vi "PotTempVI-Version3-2009.vi"() -> ()   [LabVIEW 2009]
uses:
  C/Program Files (x86)/National Instruments/LabVIEW 2014/instr.lib/Lake Shore Cryotronics 370/Lake Shore Cryotronics 370.lvlib
panel:
  in  "File Path":path
  out "Cernox Temperature 2":dbl
  out "Cernox Temperature 1":dbl
  out "Cernox Temperature 3":dbl
  out "Channel 3":cluster{dbl[], dbl[]}(graph)
  out "Channel 2":cluster{dbl[], dbl[]}(graph)
  out "Channel 1":cluster{dbl[], dbl[]}(graph)
  in  "CH1                CH2                Ch3":bool[](array[boolean])
  in  "Heater Range":u16(ring) items=["Off", "31.6 uA", "100 uA", "316 uA", "1.00 mA", "3.16 mA", "10.0 mA", "31.6 mA", "100 mA"]
  in  "Manual Output (0.000%)":dbl format="%#_13g"
  in  "(min)":dbl
  in  "(sec)":dbl
  in  "stop":bool
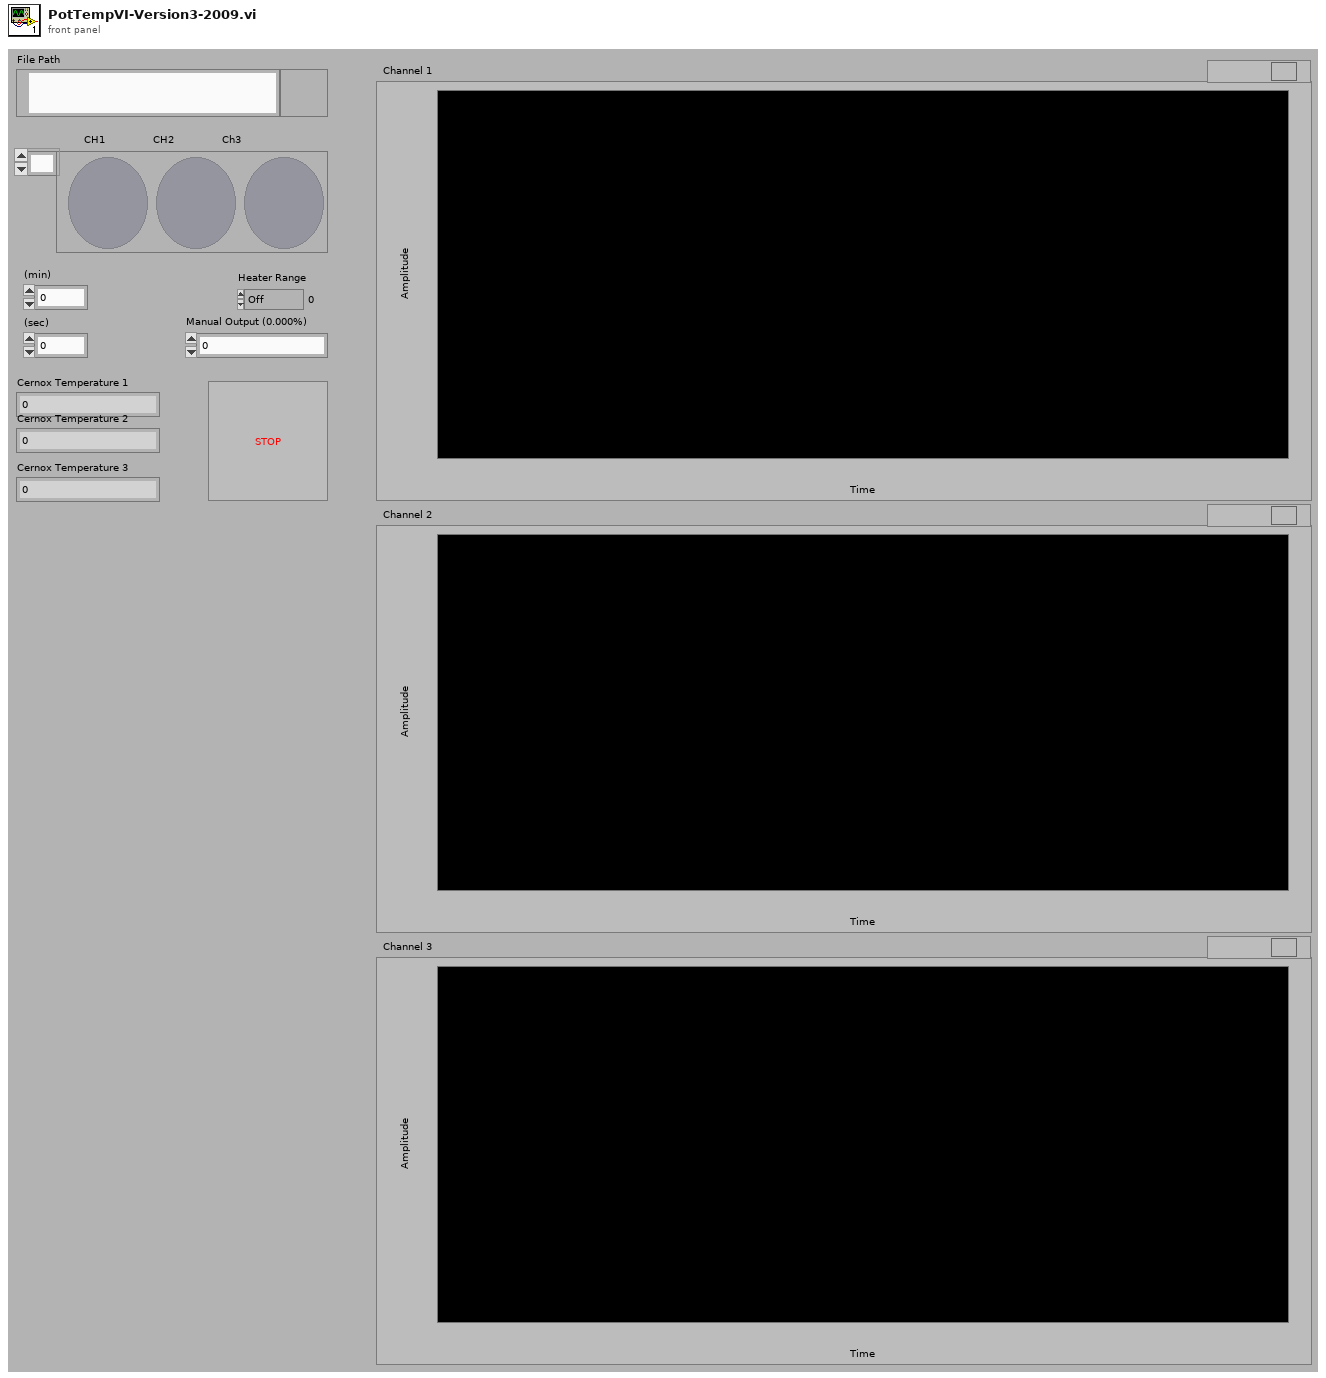
[diagram p1: front panel]
types:
  T1 = enum16{"open", "replace", "create", "open or create", "replace or create", "replace or create with confirmation"}
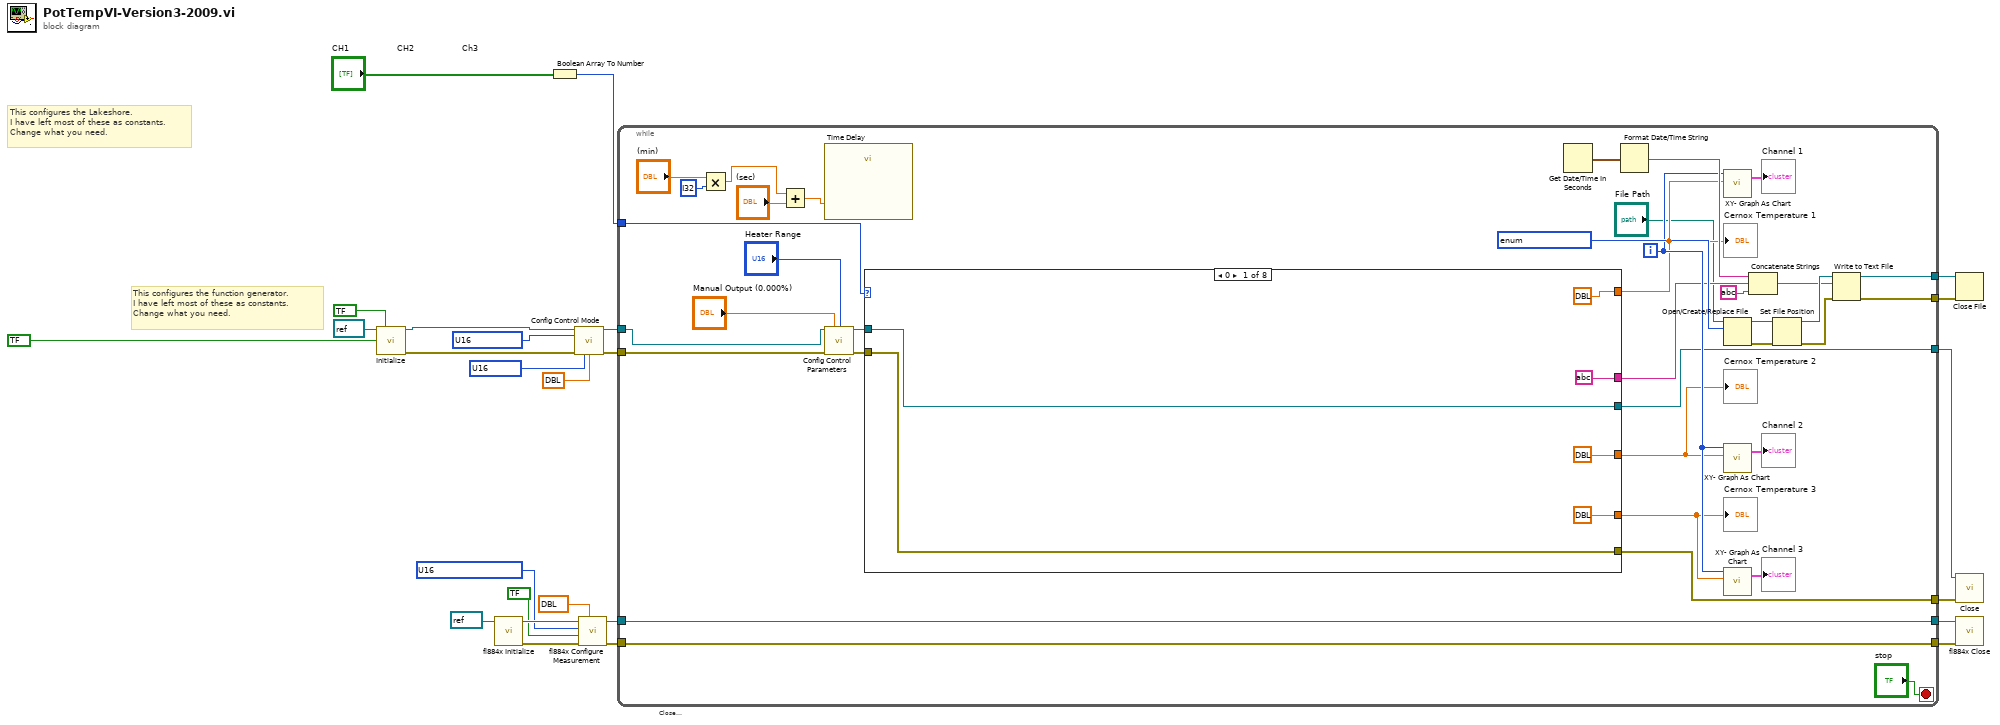
[diagram p0: block diagram]
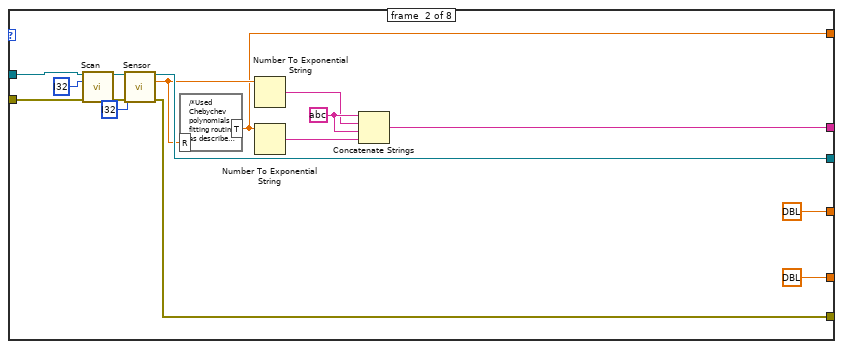
[diagram p2: hidden frame]
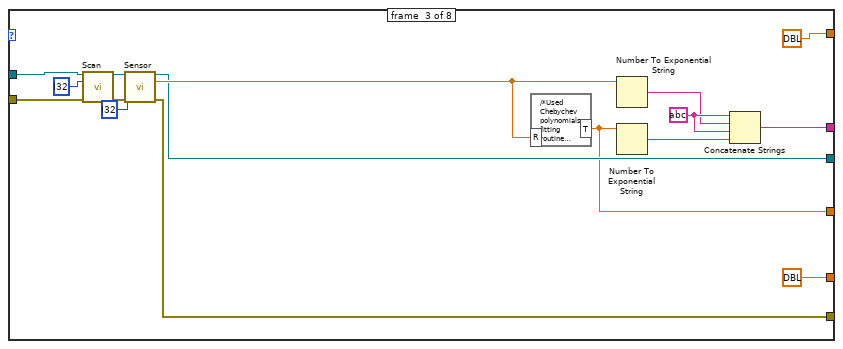
[diagram p3: hidden frame]
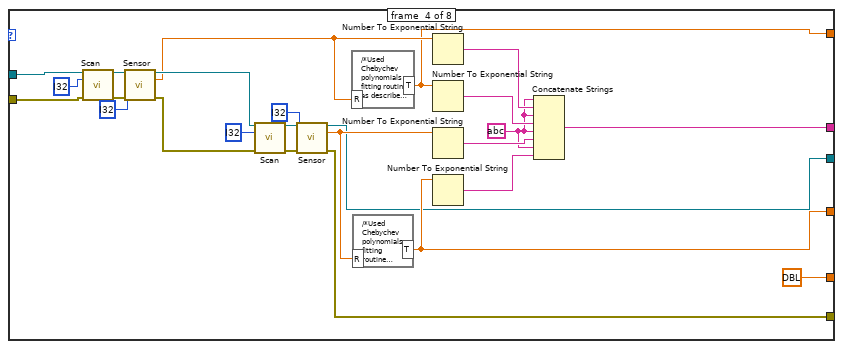
[diagram p4: hidden frame]
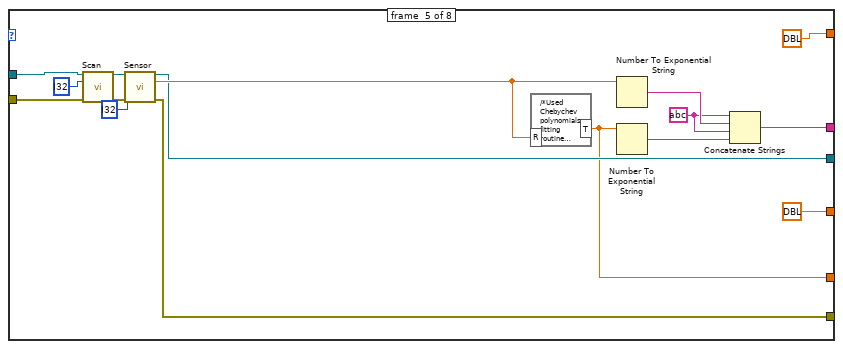
[diagram p5: hidden frame]
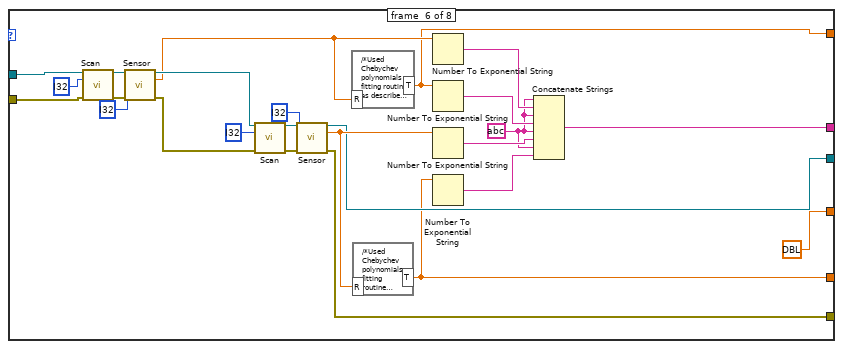
[diagram p6: hidden frame]
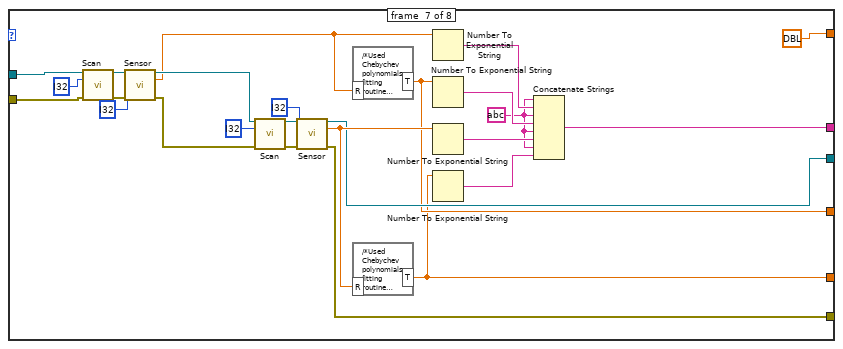
[diagram p7: hidden frame]
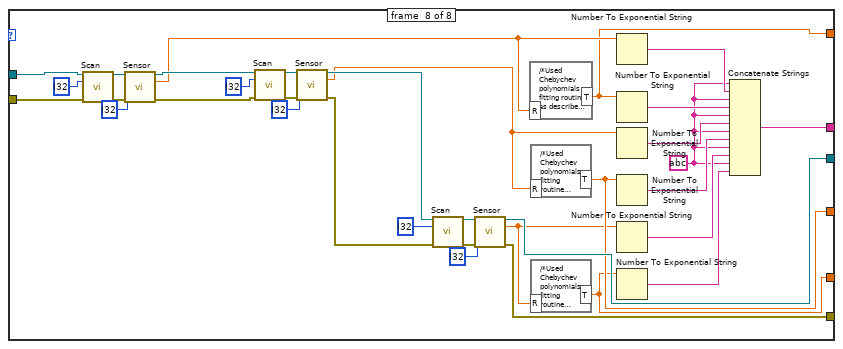
[diagram p8: hidden frame]
diagram:
  w7 = u16 ? items=["Current", "Power"] ("Heater Output Display (0: Current)")
  w9 = u16 ? items=["Closed Loop PID", "Zone Tuning", "Open Loop", "Off"] ("Control Mode (0: Closed Loop PID)")
  w23 = dbl ? items=["4.5", "5.5", "6.5"] ("Manual Resolution (5.5 Digits)")
  w24 = u16 ? items=["DC Voltage", "AC Voltage", "2 - Wire Resistance", "4 - Wire Resistance", "DC Current", "AC Current", "Frequency", "Period", "Continuity", "Diode Checking", "Temperature", "Capacitance"] ("Function (0: DC Voltage)")
  # "This configures the Lakeshore.\nI have left most of these as constants.\nChange what you need."
  # "This configures the function generator.\nI have left most of these as constants.\nChange what you need."
  # "Close Instrument."
  n1 = call "Initialize.vi"("VISA resource name"=refnum<visa-resource-name> ? ("VISA Resource Name 2"), "Reset to Default (False)"=bool ?, "Reset (True)"=bool ?) -> ("VISA resource name out"=w11:refnum<visa-resource-name>, "error out"=w10:errorcluster)  [unwired: 11 in]
  n2 = call "fl884x Initialize.vi"("VISA resource name"=refnum<visa-resource-name> ? ("VISA Resource Name")) -> ("error out"=w25:errorcluster, "VISA resource name out"=w26:refnum<visa-resource-name>)  [unwired: 9 in]
  n3 = Boolean Array To Number(Boolean array="CH1                CH2                Ch3") -> (number=w1:u32)
  n4 = call "Config Control Mode.vi"("VISA resource name"=w11, "Control Mode (0: Closed Loop PID)"=w9, "error in (no error)"=w10, "Heater Output Display (0: Current)"=w7, "Heater Resistance (100.00)"=dbl ?) -> ("VISA resource name out"=w6:refnum<visa-resource-name>, "error out"=w5:errorcluster)  [unwired: 9 in]
  n5 = call "fl884x Configure Measurement.vi"("Manual Resolution (5.5 Digits)"=w23, "error in (no error)"=w25, "Auto Range (T:Enable)"=bool ?, "Function (0: DC Voltage)"=w24, "VISA resource name"=w26) -> ("error out"=w19:errorcluster, "VISA resource name out"=w20:refnum<visa-resource-name>)  [unwired: 5 in]
  n6 = while {
    tunnel: w20 -> [w49]
    tunnel: w19 -> [w48]
    tunnel: w6 -> [w47]
    tunnel: w5 -> [w46]
    tunnel: [w49] -> w15
    tunnel: [w48] -> w18
    tunnel: [w56] -> w17
    tunnel: [w55] -> w16
    tunnel: [w35] -> w4
    tunnel: [w34] -> w3
    tunnel: w1 -> [w41]
    i -> [w36]
    stop <- "stop" stop-if-true
    n7 = Multiply(x="(min)", y=i32 ?) -> (x*y=w53:dbl)
    n8 = Add(x=w53, y="(sec)") -> (x+y=w52:dbl)
    n9 = call "Time Delay"("Delay Time (s)"=w52) -> ()  [unwired: 10 in, 1 out]
    n10 = call "Config Control Parameters.vi"("VISA resource name"=w47, "Manual Output (0.000%)"="Manual Output (0.000%)", "Heater Range (0: Off)"="Heater Range", "error in (no error)"=w46) -> ("VISA resource name out"=w40:refnum<visa-resource-name>, "error out"=w39:errorcluster)  [unwired: 10 in]
    n11 = case shown="0" w41 {
      tunnel: w40 -> [w69 w77 w93 w109 w135 w147 w174 w226]
      tunnel: w39 -> [w68 w76 w92 w108 w134 w151 w173 w225]
      tunnel: [dbl ? w71 dbl ? w104 dbl ? w145 dbl ? w197] -> w32
      tunnel: [w69 w79 w91 w107 w137 w156 w178 w214] -> w35
      tunnel: [w68 w78 w90 w106 w136 w150 w177 w213] -> w34
      tunnel: [dbl ? dbl ? w87 w110 dbl ? dbl ? w172 w206] -> w31
      tunnel: [dbl ? dbl ? dbl ? dbl ? w131 w153 w171 w202] -> w30
      tunnel: [string ? w75 w94 w112 w130 w154 w175 w199] -> w29
      frame #0 {
      }
      frame #1 {
        w85 = string ?
        n12 = call "Scan.vi"("VISA resource name"=w77, "Scan Channel (1)"=i32 ?, "error in (no error)"=w76) -> ("VISA resource name out"=w80:refnum<visa-resource-name>, "error out"=w82:errorcluster)  [unwired: 11 in]
        n13 = call "Sensor.vi"("VISA resource name"=w80, "Channel (1)"=i32 ?, "error in (no error)"=w82) -> ("VISA resource name out"=w79:refnum<visa-resource-name>, "Resistance Reading"=w72:dbl, "error out"=w78:errorcluster)  [unwired: 8 in, 2 out]
        n14 = formula code="/*Used Chebychev polynomials fitting routine\nas described in Calibration Report Description \ndocument. For future use with other thermometer, \njust replace, in all the appropriate\nranges, the Chebychev coefficients (array 'A[i]'), \nthe lower and upper boundaries for Z (variables 'ZU' \nand 'ZL'), and the numberof polynomial terms or \nfit range (variable 'range'). This information is \nfound in the data file for the corresponding \nthermometer */\n\n/*Declare variables. Used same notation\nas Lakeshore Calibration Report Description*/\n\nfloat64 Z, ZL, ZU, X, T;\nfloat64 Tc[12], A[12];\nint range, i;\nZ=log(R);\n\n\n/*Fit range 3, for R between 122.7738 and\n379.0544*/\nif(R>122.7738 && R<=379.0544)\n{\nrange=7;\nZL= 2.06767500767592;\nZU= 2.62579727581576;\nX=((Z-ZL)-(ZU-Z))/(ZU-ZL);\nA[0]=5.89345488289531E+00;\nA[1]=-6.65662879806624E+00;\nA[2]=2.58839377481062E+00;\nA[3]=-7.79761085327563E-01;\nA[4]=1.81747664835559E-01;\nA[5]=-2.85948965899305E-02;\nA[6]=3.14756394066286E-04;\nA[7]=1.58182677797188E-03;\nA[8]=-1.62769128118703E-03;\n\nTc[0]=1;\nTc[1]=X;\nT=A[0]+A[1]*X;\n\nfor(i=2; i<=range; i++)\n{\nTc[i]=2*X*Tc[i-1]-Tc[i-2];\nT=T+Tc[i]*A[i];\n}\n}\n\n/*Fit range 2, for R between 59.7368 and\n122.7738*/\nif(R> 59.7368 && R<=122.7738)\n{\nrange=7;\nZL= 1.75200116332745;\nZU= 2.11435743095945;\nX=((Z-ZL)-(ZU-Z))/(ZU-ZL);\nA[0]=4.32234727947262E+01;\nA[1]=-3.81351999747578E+01;\nA[2]=7.81449116299263E+00;\nA[3]=-8.59375474039158E-01;\nA[4]= 1.00417492862823E-01;\nA[5]=1.74498449889679E-03;\nA[6]=-1.20713645610291E-02;\nA[7]=1.63447339264850E-03;\n\nTc[0]=1;\nTc[1]=X;\nT=A[0]+A[1]*X;\n\nfor(i=2; i<=range; i++)\n{\nTc[i]=2*X*Tc[i-1]-Tc[i-2];\nT=T+Tc[i]*A[i];\n}\n}\n\n/*Fit range 1, for R between 28.7437 and\n8273.0144*/\nif(R> 28.7437 && R<=59.7368)\n{\nrange=7;\nZL= 1.45494394005744;\nZU= 1.80316018562455;\nX=((Z-ZL)-(ZU-Z))/(ZU-ZL);\nA[0]=1.78354115735659E+02;\nA[1]=-1.26988903132178E+02;\nA[2]=2.11414551345279E+01;\nA[3]=-2.87039950284064E+00;\nA[4]= 6.30799574782896E-01;\nA[5]=-1.42209214015529E-01;\nA[6]=3.09622419372907E-02;\nA[7]=-9.63520999389506E-03;\n\nTc[0]=1;\nTc[1]=X;\nT=A[0]+A[1]*X;\n\nfor(i=2; i<=range; i++)\n{\nTc[i]=2*X*Tc[i-1]-Tc[i-2];\nT=T+Tc[i]*A[i];\n}\n}"("R"=w72) -> ("T"=w71:dbl)
        n15 = Number To Exponential String(number=w72) -> (E-format string=w83:string)  [unwired: 3 in]
        n16 = Number To Exponential String(number=w71) -> (E-format string=w84:string)  [unwired: 3 in]
        n17 = Concatenate Strings(w85, w83, w85, w84) -> (w75:string)
      }
      frame #2 {
        w101 = string ?
        n18 = call "Scan.vi"("VISA resource name"=w93, "Scan Channel (1)"=i32 ?, "error in (no error)"=w92) -> ("VISA resource name out"=w95:refnum<visa-resource-name>, "error out"=w97:errorcluster)  [unwired: 11 in]
        n19 = call "Sensor.vi"("VISA resource name"=w95, "Channel (1)"=i32 ?, "error in (no error)"=w97) -> ("VISA resource name out"=w91:refnum<visa-resource-name>, "Resistance Reading"=w98:dbl, "error out"=w90:errorcluster)  [unwired: 8 in, 2 out]
        n20 = formula code="/*Used Chebychev polynomials fitting routine\nas described in Calibration Report Description \ndocument. For future use with other thermometer, \njust replace, in all the appropriate\nranges, the Chebychev coefficients (array 'A[i]'), \nthe lower and upper boundaries for Z (variables 'ZU' \nand 'ZL'), and the numberof polynomial terms or \nfit range (variable 'range'). This information is \nfound in the data file for the corresponding \nthermometer */\n\n/*Declare variables. Used same notation\nas Lakeshore Calibration Report Description*/\n\nfloat64 Z, ZL, ZU, X, T;\nfloat64 Tc[12], A[12];\nint range, i;\nZ=log(R);\n\n/*Fit range 4, for R between 27.8145 and\n55.2018*/\nif(R>=27.8145 && R<=55.2018)\n{\nrange=7;\nZL= 1.44074353015701;\nZU=1.76670659886134;\nX=((Z-ZL)-(ZU-Z))/(ZU-ZL);\nA[0]=1.82158062367373E+02;\nA[1]=-1.24663785394699E+02;\nA[2]= 1.99707471344437E+01;\nA[3]=-2.68638755066500E+00;\nA[4]=5.62902207096738E-01;\nA[5]= -1.04899492331528E-01;\nA[6]=1.47394426824740E-02;\nA[7]=-1.09663024188992E-02;\n\nTc[0]=1;\nTc[1]=X;\nT=A[0]+A[1]*X;\n\nfor(i=2; i<=range; i++)\n{\nTc[i]=2*X*Tc[i-1]-Tc[i-2];\nT=T+Tc[i]*A[i];\n}\n}\n\n/*Fit range 3, for R between 55.2018 and\n111.4842*/\nif(R>55.2018 && R<=111.4842)\n{\nrange=9;\nZL= 1.71936458773677;\nZU= 2.06940247551414;\nX=((Z-ZL)-(ZU-Z))/(ZU-ZL);\nA[0]=4.61222264729901E+01;\nA[1]=-4.01018177367225E+01;\nA[2]=8.04410401028361E+00;\nA[3]=-8.87825177741193E-01;\nA[4]= 9.46412812559081E-02;\nA[5]=1.14695723765652E-02;\nA[6]=-1.28476433375258E-02;\nA[7]=2.61003207902573E-03;\nA[8]=-1.62769128118703E-03;\nA[9]=2.14879733652881E-03;\n\nTc[0]=1;\nTc[1]=X;\nT=A[0]+A[1]*X;\n\nfor(i=2; i<=range; i++)\n{\nTc[i]=2*X*Tc[i-1]-Tc[i-2];\nT=T+Tc[i]*A[i];\n}\n}\n\n/*Fit range 2, for R between 111.4842 and\n313.6289*/\nif(R> 111.4842 && R<=313.6289)\n{\nrange=8;\nZL= 2.02806379707861;\nZU= 2.55512620740659;\nX=((Z-ZL)-(ZU-Z))/(ZU-ZL);\nA[0]=6.35009482366579E+00;\nA[1]=-7.12992063705802E+00;\nA[2]=2.72290509023981E+00;\nA[3]=-7.95127185574136E-01;\nA[4]= 1.75501651647015E-01;\nA[5]=-2.36820706103904E-02;\nA[6]=-1.48683367592906E-03;\nA[7]=2.20400453630561E-03;\nA[8]=-7.29658382785940E-04;\n\nTc[0]=1;\nTc[1]=X;\nT=A[0]+A[1]*X;\n\nfor(i=2; i<=range; i++)\n{\nTc[i]=2*X*Tc[i-1]-Tc[i-2];\nT=T+Tc[i]*A[i];\n}\n}\n\n/*Fit range 1, for R between 313.6289 and\n8273.0144*/\nif(R>  313.6289 && R<=8273.0144)\n{\nrange=11;\nZL= 2.43768275202674;\nZU= 4.08120684160154;\nX=((Z-ZL)-(ZU-Z))/(ZU-ZL);\nA[0]=5.67750174822212E-01;\nA[1]=-7.48399352555430E-01;\nA[2]=3.88178435547519E-01;\nA[3]=-1.77340445603059E-01;\nA[4]= 7.34297995027544E-02;\nA[5]=-2.89170333461975E-02;\nA[6]=1.12452775189607E-02;\nA[7]=-3.77083878348011E-03;\nA[8]=1.58754722583042E-03;\nA[9]=-1.76346768933995E-04;\nA[10]=4.11858083918786E-04;\nA[11]=3.67394984257076E-04;\n\nTc[0]=1;\nTc[1]=X;\nT=A[0]+A[1]*X;\n\nfor(i=2; i<=range; i++)\n{\nTc[i]=2*X*Tc[i-1]-Tc[i-2];\nT=T+Tc[i]*A[i];\n}\n}"("R"=w98) -> ("T"=w87:dbl)
        n21 = Number To Exponential String(number=w98) -> (E-format string=w99:string)  [unwired: 3 in]
        n22 = Number To Exponential String(number=w87) -> (E-format string=w100:string)  [unwired: 3 in]
        n23 = Concatenate Strings(w101, w99, w101, w100) -> (w94:string)
      }
      frame #3 {
        w111 = string ?
        n24 = call "Scan.vi"("VISA resource name"=w109, "Scan Channel (1)"=i32 ?, "error in (no error)"=w108) -> ("VISA resource name out"=w125:refnum<visa-resource-name>, "error out"=w124:errorcluster)  [unwired: 11 in]
        n25 = call "Sensor.vi"("VISA resource name"=w125, "Channel (1)"=i32 ?, "error in (no error)"=w124) -> ("VISA resource name out"=w122:refnum<visa-resource-name>, "Resistance Reading"=w105:dbl, "error out"=w121:errorcluster)  [unwired: 8 in, 2 out]
        n26 = call "Scan.vi"("VISA resource name"=w122, "Scan Channel (1)"=i32 ?, "error in (no error)"=w121) -> ("VISA resource name out"=w123:refnum<visa-resource-name>, "error out"=w119:errorcluster)  [unwired: 11 in]
        n27 = call "Sensor.vi"("VISA resource name"=w123, "Channel (1)"=i32 ?, "error in (no error)"=w119) -> ("VISA resource name out"=w107:refnum<visa-resource-name>, "Resistance Reading"=w116:dbl, "error out"=w106:errorcluster)  [unwired: 8 in, 2 out]
        n28 = formula code="/*Used Chebychev polynomials fitting routine\nas described in Calibration Report Description \ndocument. For future use with other thermometer, \njust replace, in all the appropriate\nranges, the Chebychev coefficients (array 'A[i]'), \nthe lower and upper boundaries for Z (variables 'ZU' \nand 'ZL'), and the numberof polynomial terms or \nfit range (variable 'range'). This information is \nfound in the data file for the corresponding \nthermometer */\n\n/*Declare variables. Used same notation\nas Lakeshore Calibration Report Description*/\n\nfloat64 Z, ZL, ZU, X, T;\nfloat64 Tc[12], A[12];\nint range, i;\nZ=log(R);\n\n\n/*Fit range 3, for R between 122.7738 and\n379.0544*/\nif(R>122.7738 && R<=379.0544)\n{\nrange=7;\nZL= 2.06767500767592;\nZU= 2.62579727581576;\nX=((Z-ZL)-(ZU-Z))/(ZU-ZL);\nA[0]=5.89345488289531E+00;\nA[1]=-6.65662879806624E+00;\nA[2]=2.58839377481062E+00;\nA[3]=-7.79761085327563E-01;\nA[4]=1.81747664835559E-01;\nA[5]=-2.85948965899305E-02;\nA[6]=3.14756394066286E-04;\nA[7]=1.58182677797188E-03;\nA[8]=-1.62769128118703E-03;\n\nTc[0]=1;\nTc[1]=X;\nT=A[0]+A[1]*X;\n\nfor(i=2; i<=range; i++)\n{\nTc[i]=2*X*Tc[i-1]-Tc[i-2];\nT=T+Tc[i]*A[i];\n}\n}\n\n/*Fit range 2, for R between 59.7368 and\n122.7738*/\nif(R> 59.7368 && R<=122.7738)\n{\nrange=7;\nZL= 1.75200116332745;\nZU= 2.11435743095945;\nX=((Z-ZL)-(ZU-Z))/(ZU-ZL);\nA[0]=4.32234727947262E+01;\nA[1]=-3.81351999747578E+01;\nA[2]=7.81449116299263E+00;\nA[3]=-8.59375474039158E-01;\nA[4]= 1.00417492862823E-01;\nA[5]=1.74498449889679E-03;\nA[6]=-1.20713645610291E-02;\nA[7]=1.63447339264850E-03;\n\nTc[0]=1;\nTc[1]=X;\nT=A[0]+A[1]*X;\n\nfor(i=2; i<=range; i++)\n{\nTc[i]=2*X*Tc[i-1]-Tc[i-2];\nT=T+Tc[i]*A[i];\n}\n}\n\n/*Fit range 1, for R between 28.7437 and\n8273.0144*/\nif(R> 28.7437 && R<=59.7368)\n{\nrange=7;\nZL= 1.45494394005744;\nZU= 1.80316018562455;\nX=((Z-ZL)-(ZU-Z))/(ZU-ZL);\nA[0]=1.78354115735659E+02;\nA[1]=-1.26988903132178E+02;\nA[2]=2.11414551345279E+01;\nA[3]=-2.87039950284064E+00;\nA[4]= 6.30799574782896E-01;\nA[5]=-1.42209214015529E-01;\nA[6]=3.09622419372907E-02;\nA[7]=-9.63520999389506E-03;\n\nTc[0]=1;\nTc[1]=X;\nT=A[0]+A[1]*X;\n\nfor(i=2; i<=range; i++)\n{\nTc[i]=2*X*Tc[i-1]-Tc[i-2];\nT=T+Tc[i]*A[i];\n}\n}"("R"=w105) -> ("T"=w104:dbl)
        n29 = formula code="/*Used Chebychev polynomials fitting routine\nas described in Calibration Report Description \ndocument. For future use with other thermometer, \njust replace, in all the appropriate\nranges, the Chebychev coefficients (array 'A[i]'), \nthe lower and upper boundaries for Z (variables 'ZU' \nand 'ZL'), and the numberof polynomial terms or \nfit range (variable 'range'). This information is \nfound in the data file for the corresponding \nthermometer */\n\n/*Declare variables. Used same notation\nas Lakeshore Calibration Report Description*/\n\nfloat64 Z, ZL, ZU, X, T;\nfloat64 Tc[12], A[12];\nint range, i;\nZ=log(R);\n\n/*Fit range 4, for R between 27.8145 and\n55.2018*/\nif(R>=27.8145 && R<=55.2018)\n{\nrange=7;\nZL= 1.44074353015701;\nZU=1.76670659886134;\nX=((Z-ZL)-(ZU-Z))/(ZU-ZL);\nA[0]=1.82158062367373E+02;\nA[1]=-1.24663785394699E+02;\nA[2]= 1.99707471344437E+01;\nA[3]=-2.68638755066500E+00;\nA[4]=5.62902207096738E-01;\nA[5]= -1.04899492331528E-01;\nA[6]=1.47394426824740E-02;\nA[7]=-1.09663024188992E-02;\n\nTc[0]=1;\nTc[1]=X;\nT=A[0]+A[1]*X;\n\nfor(i=2; i<=range; i++)\n{\nTc[i]=2*X*Tc[i-1]-Tc[i-2];\nT=T+Tc[i]*A[i];\n}\n}\n\n/*Fit range 3, for R between 55.2018 and\n111.4842*/\nif(R>55.2018 && R<=111.4842)\n{\nrange=9;\nZL= 1.71936458773677;\nZU= 2.06940247551414;\nX=((Z-ZL)-(ZU-Z))/(ZU-ZL);\nA[0]=4.61222264729901E+01;\nA[1]=-4.01018177367225E+01;\nA[2]=8.04410401028361E+00;\nA[3]=-8.87825177741193E-01;\nA[4]= 9.46412812559081E-02;\nA[5]=1.14695723765652E-02;\nA[6]=-1.28476433375258E-02;\nA[7]=2.61003207902573E-03;\nA[8]=-1.62769128118703E-03;\nA[9]=2.14879733652881E-03;\n\nTc[0]=1;\nTc[1]=X;\nT=A[0]+A[1]*X;\n\nfor(i=2; i<=range; i++)\n{\nTc[i]=2*X*Tc[i-1]-Tc[i-2];\nT=T+Tc[i]*A[i];\n}\n}\n\n/*Fit range 2, for R between 111.4842 and\n313.6289*/\nif(R> 111.4842 && R<=313.6289)\n{\nrange=8;\nZL= 2.02806379707861;\nZU= 2.55512620740659;\nX=((Z-ZL)-(ZU-Z))/(ZU-ZL);\nA[0]=6.35009482366579E+00;\nA[1]=-7.12992063705802E+00;\nA[2]=2.72290509023981E+00;\nA[3]=-7.95127185574136E-01;\nA[4]= 1.75501651647015E-01;\nA[5]=-2.36820706103904E-02;\nA[6]=-1.48683367592906E-03;\nA[7]=2.20400453630561E-03;\nA[8]=-7.29658382785940E-04;\n\nTc[0]=1;\nTc[1]=X;\nT=A[0]+A[1]*X;\n\nfor(i=2; i<=range; i++)\n{\nTc[i]=2*X*Tc[i-1]-Tc[i-2];\nT=T+Tc[i]*A[i];\n}\n}\n\n/*Fit range 1, for R between 313.6289 and\n8273.0144*/\nif(R>  313.6289 && R<=8273.0144)\n{\nrange=11;\nZL= 2.43768275202674;\nZU= 4.08120684160154;\nX=((Z-ZL)-(ZU-Z))/(ZU-ZL);\nA[0]=5.67750174822212E-01;\nA[1]=-7.48399352555430E-01;\nA[2]=3.88178435547519E-01;\nA[3]=-1.77340445603059E-01;\nA[4]= 7.34297995027544E-02;\nA[5]=-2.89170333461975E-02;\nA[6]=1.12452775189607E-02;\nA[7]=-3.77083878348011E-03;\nA[8]=1.58754722583042E-03;\nA[9]=-1.76346768933995E-04;\nA[10]=4.11858083918786E-04;\nA[11]=3.67394984257076E-04;\n\nTc[0]=1;\nTc[1]=X;\nT=A[0]+A[1]*X;\n\nfor(i=2; i<=range; i++)\n{\nTc[i]=2*X*Tc[i-1]-Tc[i-2];\nT=T+Tc[i]*A[i];\n}\n}"("R"=w116) -> ("T"=w110:dbl)
        n30 = Number To Exponential String(number=w105) -> (E-format string=w118:string)  [unwired: 3 in]
        n31 = Number To Exponential String(number=w104) -> (E-format string=w117:string)  [unwired: 3 in]
        n32 = Number To Exponential String(number=w116) -> (E-format string=w115:string)  [unwired: 3 in]
        n33 = Number To Exponential String(number=w110) -> (E-format string=w114:string)  [unwired: 3 in]
        n34 = Concatenate Strings(w111, w118, w111, w117, w111, w115, w111, w114) -> (w112:string)
      }
      frame #4 {
        w128 = string ?
        n35 = call "Scan.vi"("VISA resource name"=w135, "Scan Channel (1)"=i32 ?, "error in (no error)"=w134) -> ("VISA resource name out"=w142:refnum<visa-resource-name>, "error out"=w140:errorcluster)  [unwired: 11 in]
        n36 = call "Sensor.vi"("VISA resource name"=w142, "Channel (1)"=i32 ?, "error in (no error)"=w140) -> ("VISA resource name out"=w137:refnum<visa-resource-name>, "Resistance Reading"=w139:dbl, "error out"=w136:errorcluster)  [unwired: 8 in, 2 out]
        n37 = formula code="/*Used Chebychev polynomials fitting routine\nas described in Calibration Report Description \ndocument. For future use with other thermometer, \njust replace, in all the appropriate\nranges, the Chebychev coefficients (array 'A[i]'), \nthe lower and upper boundaries for Z (variables 'ZU' \nand 'ZL'), and the numberof polynomial terms or \nfit range (variable 'range'). This information is \nfound in the data file for the corresponding \nthermometer */\n\n/*Declare variables. Used same notation\nas Lakeshore Calibration Report Description*/\n\nfloat64 Z, ZL, ZU, X, T;\nfloat64 Tc[12], A[12];\nint range, i;\nZ=log(R);\n\n/*Fit range 4, for R between 27.8145 and\n55.2018*/\nif(R>=27.8145 && R<=55.2018)\n{\nrange=7;\nZL= 1.44074353015701;\nZU=1.76670659886134;\nX=((Z-ZL)-(ZU-Z))/(ZU-ZL);\nA[0]=1.82158062367373E+02;\nA[1]=-1.24663785394699E+02;\nA[2]= 1.99707471344437E+01;\nA[3]=-2.68638755066500E+00;\nA[4]=5.62902207096738E-01;\nA[5]= -1.04899492331528E-01;\nA[6]=1.47394426824740E-02;\nA[7]=-1.09663024188992E-02;\n\nTc[0]=1;\nTc[1]=X;\nT=A[0]+A[1]*X;\n\nfor(i=2; i<=range; i++)\n{\nTc[i]=2*X*Tc[i-1]-Tc[i-2];\nT=T+Tc[i]*A[i];\n}\n}\n\n/*Fit range 3, for R between 55.2018 and\n111.4842*/\nif(R>55.2018 && R<=111.4842)\n{\nrange=9;\nZL= 1.71936458773677;\nZU= 2.06940247551414;\nX=((Z-ZL)-(ZU-Z))/(ZU-ZL);\nA[0]=4.61222264729901E+01;\nA[1]=-4.01018177367225E+01;\nA[2]=8.04410401028361E+00;\nA[3]=-8.87825177741193E-01;\nA[4]= 9.46412812559081E-02;\nA[5]=1.14695723765652E-02;\nA[6]=-1.28476433375258E-02;\nA[7]=2.61003207902573E-03;\nA[8]=-1.62769128118703E-03;\nA[9]=2.14879733652881E-03;\n\nTc[0]=1;\nTc[1]=X;\nT=A[0]+A[1]*X;\n\nfor(i=2; i<=range; i++)\n{\nTc[i]=2*X*Tc[i-1]-Tc[i-2];\nT=T+Tc[i]*A[i];\n}\n}\n\n/*Fit range 2, for R between 111.4842 and\n313.6289*/\nif(R> 111.4842 && R<=313.6289)\n{\nrange=8;\nZL= 2.02806379707861;\nZU= 2.55512620740659;\nX=((Z-ZL)-(ZU-Z))/(ZU-ZL);\nA[0]=6.35009482366579E+00;\nA[1]=-7.12992063705802E+00;\nA[2]=2.72290509023981E+00;\nA[3]=-7.95127185574136E-01;\nA[4]= 1.75501651647015E-01;\nA[5]=-2.36820706103904E-02;\nA[6]=-1.48683367592906E-03;\nA[7]=2.20400453630561E-03;\nA[8]=-7.29658382785940E-04;\n\nTc[0]=1;\nTc[1]=X;\nT=A[0]+A[1]*X;\n\nfor(i=2; i<=range; i++)\n{\nTc[i]=2*X*Tc[i-1]-Tc[i-2];\nT=T+Tc[i]*A[i];\n}\n}\n\n/*Fit range 1, for R between 313.6289 and\n8273.0144*/\nif(R>  313.6289 && R<=8273.0144)\n{\nrange=11;\nZL= 2.43768275202674;\nZU= 4.08120684160154;\nX=((Z-ZL)-(ZU-Z))/(ZU-ZL);\nA[0]=5.67750174822212E-01;\nA[1]=-7.48399352555430E-01;\nA[2]=3.88178435547519E-01;\nA[3]=-1.77340445603059E-01;\nA[4]= 7.34297995027544E-02;\nA[5]=-2.89170333461975E-02;\nA[6]=1.12452775189607E-02;\nA[7]=-3.77083878348011E-03;\nA[8]=1.58754722583042E-03;\nA[9]=-1.76346768933995E-04;\nA[10]=4.11858083918786E-04;\nA[11]=3.67394984257076E-04;\n\nTc[0]=1;\nTc[1]=X;\nT=A[0]+A[1]*X;\n\nfor(i=2; i<=range; i++)\n{\nTc[i]=2*X*Tc[i-1]-Tc[i-2];\nT=T+Tc[i]*A[i];\n}\n}"("R"=w139) -> ("T"=w131:dbl)
        n38 = Number To Exponential String(number=w139) -> (E-format string=w138:string)  [unwired: 3 in]
        n39 = Number To Exponential String(number=w131) -> (E-format string=w129:string)  [unwired: 3 in]
        n40 = Concatenate Strings(w128, w138, w128, w129) -> (w130:string)
      }
      frame #5 {
        w157 = string ?
        n41 = call "Scan.vi"("VISA resource name"=w147, "Scan Channel (1)"=i32 ?, "error in (no error)"=w151) -> ("VISA resource name out"=w166:refnum<visa-resource-name>, "error out"=w165:errorcluster)  [unwired: 11 in]
        n42 = call "Sensor.vi"("VISA resource name"=w166, "Channel (1)"=i32 ?, "error in (no error)"=w165) -> ("VISA resource name out"=w149:refnum<visa-resource-name>, "Resistance Reading"=w146:dbl, "error out"=w148:errorcluster)  [unwired: 8 in, 2 out]
        n43 = call "Scan.vi"("VISA resource name"=w149, "Scan Channel (1)"=i32 ?, "error in (no error)"=w148) -> ("VISA resource name out"=w164:refnum<visa-resource-name>, "error out"=w162:errorcluster)  [unwired: 11 in]
        n44 = call "Sensor.vi"("VISA resource name"=w164, "Channel (1)"=i32 ?, "error in (no error)"=w162) -> ("VISA resource name out"=w156:refnum<visa-resource-name>, "Resistance Reading"=w159:dbl, "error out"=w150:errorcluster)  [unwired: 8 in, 2 out]
        n45 = formula code="/*Used Chebychev polynomials fitting routine\nas described in Calibration Report Description \ndocument. For future use with other thermometer, \njust replace, in all the appropriate\nranges, the Chebychev coefficients (array 'A[i]'), \nthe lower and upper boundaries for Z (variables 'ZU' \nand 'ZL'), and the numberof polynomial terms or \nfit range (variable 'range'). This information is \nfound in the data file for the corresponding \nthermometer */\n\n/*Declare variables. Used same notation\nas Lakeshore Calibration Report Description*/\n\nfloat64 Z, ZL, ZU, X, T;\nfloat64 Tc[12], A[12];\nint range, i;\nZ=log(R);\n\n\n/*Fit range 3, for R between 122.7738 and\n379.0544*/\nif(R>122.7738 && R<=379.0544)\n{\nrange=7;\nZL= 2.06767500767592;\nZU= 2.62579727581576;\nX=((Z-ZL)-(ZU-Z))/(ZU-ZL);\nA[0]=5.89345488289531E+00;\nA[1]=-6.65662879806624E+00;\nA[2]=2.58839377481062E+00;\nA[3]=-7.79761085327563E-01;\nA[4]=1.81747664835559E-01;\nA[5]=-2.85948965899305E-02;\nA[6]=3.14756394066286E-04;\nA[7]=1.58182677797188E-03;\nA[8]=-1.62769128118703E-03;\n\nTc[0]=1;\nTc[1]=X;\nT=A[0]+A[1]*X;\n\nfor(i=2; i<=range; i++)\n{\nTc[i]=2*X*Tc[i-1]-Tc[i-2];\nT=T+Tc[i]*A[i];\n}\n}\n\n/*Fit range 2, for R between 59.7368 and\n122.7738*/\nif(R> 59.7368 && R<=122.7738)\n{\nrange=7;\nZL= 1.75200116332745;\nZU= 2.11435743095945;\nX=((Z-ZL)-(ZU-Z))/(ZU-ZL);\nA[0]=4.32234727947262E+01;\nA[1]=-3.81351999747578E+01;\nA[2]=7.81449116299263E+00;\nA[3]=-8.59375474039158E-01;\nA[4]= 1.00417492862823E-01;\nA[5]=1.74498449889679E-03;\nA[6]=-1.20713645610291E-02;\nA[7]=1.63447339264850E-03;\n\nTc[0]=1;\nTc[1]=X;\nT=A[0]+A[1]*X;\n\nfor(i=2; i<=range; i++)\n{\nTc[i]=2*X*Tc[i-1]-Tc[i-2];\nT=T+Tc[i]*A[i];\n}\n}\n\n/*Fit range 1, for R between 28.7437 and\n8273.0144*/\nif(R> 28.7437 && R<=59.7368)\n{\nrange=7;\nZL= 1.45494394005744;\nZU= 1.80316018562455;\nX=((Z-ZL)-(ZU-Z))/(ZU-ZL);\nA[0]=1.78354115735659E+02;\nA[1]=-1.26988903132178E+02;\nA[2]=2.11414551345279E+01;\nA[3]=-2.87039950284064E+00;\nA[4]= 6.30799574782896E-01;\nA[5]=-1.42209214015529E-01;\nA[6]=3.09622419372907E-02;\nA[7]=-9.63520999389506E-03;\n\nTc[0]=1;\nTc[1]=X;\nT=A[0]+A[1]*X;\n\nfor(i=2; i<=range; i++)\n{\nTc[i]=2*X*Tc[i-1]-Tc[i-2];\nT=T+Tc[i]*A[i];\n}\n}"("R"=w146) -> ("T"=w145:dbl)
        n46 = formula code="/*Used Chebychev polynomials fitting routine\nas described in Calibration Report Description \ndocument. For future use with other thermometer, \njust replace, in all the appropriate\nranges, the Chebychev coefficients (array 'A[i]'), \nthe lower and upper boundaries for Z (variables 'ZU' \nand 'ZL'), and the numberof polynomial terms or \nfit range (variable 'range'). This information is \nfound in the data file for the corresponding \nthermometer */\n\n/*Declare variables. Used same notation\nas Lakeshore Calibration Report Description*/\n\nfloat64 Z, ZL, ZU, X, T;\nfloat64 Tc[12], A[12];\nint range, i;\nZ=log(R);\n\n/*Fit range 4, for R between 27.8145 and\n55.2018*/\nif(R>=27.8145 && R<=55.2018)\n{\nrange=7;\nZL= 1.44074353015701;\nZU=1.76670659886134;\nX=((Z-ZL)-(ZU-Z))/(ZU-ZL);\nA[0]=1.82158062367373E+02;\nA[1]=-1.24663785394699E+02;\nA[2]= 1.99707471344437E+01;\nA[3]=-2.68638755066500E+00;\nA[4]=5.62902207096738E-01;\nA[5]= -1.04899492331528E-01;\nA[6]=1.47394426824740E-02;\nA[7]=-1.09663024188992E-02;\n\nTc[0]=1;\nTc[1]=X;\nT=A[0]+A[1]*X;\n\nfor(i=2; i<=range; i++)\n{\nTc[i]=2*X*Tc[i-1]-Tc[i-2];\nT=T+Tc[i]*A[i];\n}\n}\n\n/*Fit range 3, for R between 55.2018 and\n111.4842*/\nif(R>55.2018 && R<=111.4842)\n{\nrange=9;\nZL= 1.71936458773677;\nZU= 2.06940247551414;\nX=((Z-ZL)-(ZU-Z))/(ZU-ZL);\nA[0]=4.61222264729901E+01;\nA[1]=-4.01018177367225E+01;\nA[2]=8.04410401028361E+00;\nA[3]=-8.87825177741193E-01;\nA[4]= 9.46412812559081E-02;\nA[5]=1.14695723765652E-02;\nA[6]=-1.28476433375258E-02;\nA[7]=2.61003207902573E-03;\nA[8]=-1.62769128118703E-03;\nA[9]=2.14879733652881E-03;\n\nTc[0]=1;\nTc[1]=X;\nT=A[0]+A[1]*X;\n\nfor(i=2; i<=range; i++)\n{\nTc[i]=2*X*Tc[i-1]-Tc[i-2];\nT=T+Tc[i]*A[i];\n}\n}\n\n/*Fit range 2, for R between 111.4842 and\n313.6289*/\nif(R> 111.4842 && R<=313.6289)\n{\nrange=8;\nZL= 2.02806379707861;\nZU= 2.55512620740659;\nX=((Z-ZL)-(ZU-Z))/(ZU-ZL);\nA[0]=6.35009482366579E+00;\nA[1]=-7.12992063705802E+00;\nA[2]=2.72290509023981E+00;\nA[3]=-7.95127185574136E-01;\nA[4]= 1.75501651647015E-01;\nA[5]=-2.36820706103904E-02;\nA[6]=-1.48683367592906E-03;\nA[7]=2.20400453630561E-03;\nA[8]=-7.29658382785940E-04;\n\nTc[0]=1;\nTc[1]=X;\nT=A[0]+A[1]*X;\n\nfor(i=2; i<=range; i++)\n{\nTc[i]=2*X*Tc[i-1]-Tc[i-2];\nT=T+Tc[i]*A[i];\n}\n}\n\n/*Fit range 1, for R between 313.6289 and\n8273.0144*/\nif(R>  313.6289 && R<=8273.0144)\n{\nrange=11;\nZL= 2.43768275202674;\nZU= 4.08120684160154;\nX=((Z-ZL)-(ZU-Z))/(ZU-ZL);\nA[0]=5.67750174822212E-01;\nA[1]=-7.48399352555430E-01;\nA[2]=3.88178435547519E-01;\nA[3]=-1.77340445603059E-01;\nA[4]= 7.34297995027544E-02;\nA[5]=-2.89170333461975E-02;\nA[6]=1.12452775189607E-02;\nA[7]=-3.77083878348011E-03;\nA[8]=1.58754722583042E-03;\nA[9]=-1.76346768933995E-04;\nA[10]=4.11858083918786E-04;\nA[11]=3.67394984257076E-04;\n\nTc[0]=1;\nTc[1]=X;\nT=A[0]+A[1]*X;\n\nfor(i=2; i<=range; i++)\n{\nTc[i]=2*X*Tc[i-1]-Tc[i-2];\nT=T+Tc[i]*A[i];\n}\n}"("R"=w159) -> ("T"=w153:dbl)
        n47 = Number To Exponential String(number=w146) -> (E-format string=w161:string)  [unwired: 3 in]
        n48 = Number To Exponential String(number=w145) -> (E-format string=w160:string)  [unwired: 3 in]
        n49 = Number To Exponential String(number=w159) -> (E-format string=w158:string)  [unwired: 3 in]
        n50 = Number To Exponential String(number=w153) -> (E-format string=w155:string)  [unwired: 3 in]
        n51 = Concatenate Strings(w157, w161, w157, w160, w157, w158, w157, w155) -> (w154:string)
      }
      frame #6 {
        w179 = string ?
        n52 = call "Scan.vi"("VISA resource name"=w174, "Scan Channel (1)"=i32 ?, "error in (no error)"=w173) -> ("VISA resource name out"=w192:refnum<visa-resource-name>, "error out"=w188:errorcluster)  [unwired: 11 in]
        n53 = call "Sensor.vi"("VISA resource name"=w192, "Channel (1)"=i32 ?, "error in (no error)"=w188) -> ("VISA resource name out"=w187:refnum<visa-resource-name>, "Resistance Reading"=w184:dbl, "error out"=w186:errorcluster)  [unwired: 8 in, 2 out]
        n54 = call "Scan.vi"("VISA resource name"=w187, "Scan Channel (1)"=i32 ?, "error in (no error)"=w186) -> ("VISA resource name out"=w190:refnum<visa-resource-name>, "error out"=w185:errorcluster)  [unwired: 11 in]
        n55 = call "Sensor.vi"("VISA resource name"=w190, "Channel (1)"=i32 ?, "error in (no error)"=w185) -> ("VISA resource name out"=w178:refnum<visa-resource-name>, "Resistance Reading"=w181:dbl, "error out"=w177:errorcluster)  [unwired: 8 in, 2 out]
        n56 = formula code="/*Used Chebychev polynomials fitting routine\nas described in Calibration Report Description \ndocument. For future use with other thermometer, \njust replace, in all the appropriate\nranges, the Chebychev coefficients (array 'A[i]'), \nthe lower and upper boundaries for Z (variables 'ZU' \nand 'ZL'), and the numberof polynomial terms or \nfit range (variable 'range'). This information is \nfound in the data file for the corresponding \nthermometer */\n\n/*Declare variables. Used same notation\nas Lakeshore Calibration Report Description*/\n\nfloat64 Z, ZL, ZU, X, T;\nfloat64 Tc[12], A[12];\nint range, i;\nZ=log(R);\n\n/*Fit range 4, for R between 27.8145 and\n55.2018*/\nif(R>=27.8145 && R<=55.2018)\n{\nrange=7;\nZL= 1.44074353015701;\nZU=1.76670659886134;\nX=((Z-ZL)-(ZU-Z))/(ZU-ZL);\nA[0]=1.82158062367373E+02;\nA[1]=-1.24663785394699E+02;\nA[2]= 1.99707471344437E+01;\nA[3]=-2.68638755066500E+00;\nA[4]=5.62902207096738E-01;\nA[5]= -1.04899492331528E-01;\nA[6]=1.47394426824740E-02;\nA[7]=-1.09663024188992E-02;\n\nTc[0]=1;\nTc[1]=X;\nT=A[0]+A[1]*X;\n\nfor(i=2; i<=range; i++)\n{\nTc[i]=2*X*Tc[i-1]-Tc[i-2];\nT=T+Tc[i]*A[i];\n}\n}\n\n/*Fit range 3, for R between 55.2018 and\n111.4842*/\nif(R>55.2018 && R<=111.4842)\n{\nrange=9;\nZL= 1.71936458773677;\nZU= 2.06940247551414;\nX=((Z-ZL)-(ZU-Z))/(ZU-ZL);\nA[0]=4.61222264729901E+01;\nA[1]=-4.01018177367225E+01;\nA[2]=8.04410401028361E+00;\nA[3]=-8.87825177741193E-01;\nA[4]= 9.46412812559081E-02;\nA[5]=1.14695723765652E-02;\nA[6]=-1.28476433375258E-02;\nA[7]=2.61003207902573E-03;\nA[8]=-1.62769128118703E-03;\nA[9]=2.14879733652881E-03;\n\nTc[0]=1;\nTc[1]=X;\nT=A[0]+A[1]*X;\n\nfor(i=2; i<=range; i++)\n{\nTc[i]=2*X*Tc[i-1]-Tc[i-2];\nT=T+Tc[i]*A[i];\n}\n}\n\n/*Fit range 2, for R between 111.4842 and\n313.6289*/\nif(R> 111.4842 && R<=313.6289)\n{\nrange=8;\nZL= 2.02806379707861;\nZU= 2.55512620740659;\nX=((Z-ZL)-(ZU-Z))/(ZU-ZL);\nA[0]=6.35009482366579E+00;\nA[1]=-7.12992063705802E+00;\nA[2]=2.72290509023981E+00;\nA[3]=-7.95127185574136E-01;\nA[4]= 1.75501651647015E-01;\nA[5]=-2.36820706103904E-02;\nA[6]=-1.48683367592906E-03;\nA[7]=2.20400453630561E-03;\nA[8]=-7.29658382785940E-04;\n\nTc[0]=1;\nTc[1]=X;\nT=A[0]+A[1]*X;\n\nfor(i=2; i<=range; i++)\n{\nTc[i]=2*X*Tc[i-1]-Tc[i-2];\nT=T+Tc[i]*A[i];\n}\n}\n\n/*Fit range 1, for R between 313.6289 and\n8273.0144*/\nif(R>  313.6289 && R<=8273.0144)\n{\nrange=11;\nZL= 2.43768275202674;\nZU= 4.08120684160154;\nX=((Z-ZL)-(ZU-Z))/(ZU-ZL);\nA[0]=5.67750174822212E-01;\nA[1]=-7.48399352555430E-01;\nA[2]=3.88178435547519E-01;\nA[3]=-1.77340445603059E-01;\nA[4]= 7.34297995027544E-02;\nA[5]=-2.89170333461975E-02;\nA[6]=1.12452775189607E-02;\nA[7]=-3.77083878348011E-03;\nA[8]=1.58754722583042E-03;\nA[9]=-1.76346768933995E-04;\nA[10]=4.11858083918786E-04;\nA[11]=3.67394984257076E-04;\n\nTc[0]=1;\nTc[1]=X;\nT=A[0]+A[1]*X;\n\nfor(i=2; i<=range; i++)\n{\nTc[i]=2*X*Tc[i-1]-Tc[i-2];\nT=T+Tc[i]*A[i];\n}\n}"("R"=w184) -> ("T"=w172:dbl)
        n57 = formula code="/*Used Chebychev polynomials fitting routine\nas described in Calibration Report Description \ndocument. For future use with other thermometer, \njust replace, in all the appropriate\nranges, the Chebychev coefficients (array 'A[i]'), \nthe lower and upper boundaries for Z (variables 'ZU' \nand 'ZL'), and the numberof polynomial terms or \nfit range (variable 'range'). This information is \nfound in the data file for the corresponding \nthermometer */\n\n/*Declare variables. Used same notation\nas Lakeshore Calibration Report Description*/\n\nfloat64 Z, ZL, ZU, X, T;\nfloat64 Tc[12], A[12];\nint range, i;\nZ=log(R);\n\n/*Fit range 4, for R between 27.8145 and\n55.2018*/\nif(R>=27.8145 && R<=55.2018)\n{\nrange=7;\nZL= 1.44074353015701;\nZU=1.76670659886134;\nX=((Z-ZL)-(ZU-Z))/(ZU-ZL);\nA[0]=1.82158062367373E+02;\nA[1]=-1.24663785394699E+02;\nA[2]= 1.99707471344437E+01;\nA[3]=-2.68638755066500E+00;\nA[4]=5.62902207096738E-01;\nA[5]= -1.04899492331528E-01;\nA[6]=1.47394426824740E-02;\nA[7]=-1.09663024188992E-02;\n\nTc[0]=1;\nTc[1]=X;\nT=A[0]+A[1]*X;\n\nfor(i=2; i<=range; i++)\n{\nTc[i]=2*X*Tc[i-1]-Tc[i-2];\nT=T+Tc[i]*A[i];\n}\n}\n\n/*Fit range 3, for R between 55.2018 and\n111.4842*/\nif(R>55.2018 && R<=111.4842)\n{\nrange=9;\nZL= 1.71936458773677;\nZU= 2.06940247551414;\nX=((Z-ZL)-(ZU-Z))/(ZU-ZL);\nA[0]=4.61222264729901E+01;\nA[1]=-4.01018177367225E+01;\nA[2]=8.04410401028361E+00;\nA[3]=-8.87825177741193E-01;\nA[4]= 9.46412812559081E-02;\nA[5]=1.14695723765652E-02;\nA[6]=-1.28476433375258E-02;\nA[7]=2.61003207902573E-03;\nA[8]=-1.62769128118703E-03;\nA[9]=2.14879733652881E-03;\n\nTc[0]=1;\nTc[1]=X;\nT=A[0]+A[1]*X;\n\nfor(i=2; i<=range; i++)\n{\nTc[i]=2*X*Tc[i-1]-Tc[i-2];\nT=T+Tc[i]*A[i];\n}\n}\n\n/*Fit range 2, for R between 111.4842 and\n313.6289*/\nif(R> 111.4842 && R<=313.6289)\n{\nrange=8;\nZL= 2.02806379707861;\nZU= 2.55512620740659;\nX=((Z-ZL)-(ZU-Z))/(ZU-ZL);\nA[0]=6.35009482366579E+00;\nA[1]=-7.12992063705802E+00;\nA[2]=2.72290509023981E+00;\nA[3]=-7.95127185574136E-01;\nA[4]= 1.75501651647015E-01;\nA[5]=-2.36820706103904E-02;\nA[6]=-1.48683367592906E-03;\nA[7]=2.20400453630561E-03;\nA[8]=-7.29658382785940E-04;\n\nTc[0]=1;\nTc[1]=X;\nT=A[0]+A[1]*X;\n\nfor(i=2; i<=range; i++)\n{\nTc[i]=2*X*Tc[i-1]-Tc[i-2];\nT=T+Tc[i]*A[i];\n}\n}\n\n/*Fit range 1, for R between 313.6289 and\n8273.0144*/\nif(R>  313.6289 && R<=8273.0144)\n{\nrange=11;\nZL= 2.43768275202674;\nZU= 4.08120684160154;\nX=((Z-ZL)-(ZU-Z))/(ZU-ZL);\nA[0]=5.67750174822212E-01;\nA[1]=-7.48399352555430E-01;\nA[2]=3.88178435547519E-01;\nA[3]=-1.77340445603059E-01;\nA[4]= 7.34297995027544E-02;\nA[5]=-2.89170333461975E-02;\nA[6]=1.12452775189607E-02;\nA[7]=-3.77083878348011E-03;\nA[8]=1.58754722583042E-03;\nA[9]=-1.76346768933995E-04;\nA[10]=4.11858083918786E-04;\nA[11]=3.67394984257076E-04;\n\nTc[0]=1;\nTc[1]=X;\nT=A[0]+A[1]*X;\n\nfor(i=2; i<=range; i++)\n{\nTc[i]=2*X*Tc[i-1]-Tc[i-2];\nT=T+Tc[i]*A[i];\n}\n}"("R"=w181) -> ("T"=w171:dbl)
        n58 = Number To Exponential String(number=w184) -> (E-format string=w183:string)  [unwired: 3 in]
        n59 = Number To Exponential String(number=w172) -> (E-format string=w182:string)  [unwired: 3 in]
        n60 = Number To Exponential String(number=w181) -> (E-format string=w180:string)  [unwired: 3 in]
        n61 = Number To Exponential String(number=w171) -> (E-format string=w176:string)  [unwired: 3 in]
        n62 = Concatenate Strings(w179, w183, w179, w182, w179, w180, w179, w176) -> (w175:string)
      }
      frame #7 {
        w201 = string ?
        n63 = call "Scan.vi"("VISA resource name"=w226, "Scan Channel (1)"=i32 ?, "error in (no error)"=w225) -> ("VISA resource name out"=w223:refnum<visa-resource-name>, "error out"=w222:errorcluster)  [unwired: 11 in]
        n64 = call "Sensor.vi"("VISA resource name"=w223, "Channel (1)"=i32 ?, "error in (no error)"=w222) -> ("VISA resource name out"=w220:refnum<visa-resource-name>, "Resistance Reading"=w198:dbl, "error out"=w219:errorcluster)  [unwired: 8 in, 2 out]
        n65 = call "Scan.vi"("VISA resource name"=w220, "Scan Channel (1)"=i32 ?, "error in (no error)"=w219) -> ("VISA resource name out"=w221:refnum<visa-resource-name>, "error out"=w215:errorcluster)  [unwired: 11 in]
        n66 = call "Sensor.vi"("VISA resource name"=w221, "Channel (1)"=i32 ?, "error in (no error)"=w215) -> ("VISA resource name out"=w212:refnum<visa-resource-name>, "Resistance Reading"=w208:dbl, "error out"=w195:errorcluster)  [unwired: 8 in, 2 out]
        n67 = call "Scan.vi"("VISA resource name"=w212, "Scan Channel (1)"=i32 ?, "error in (no error)"=w195) -> ("VISA resource name out"=w217:refnum<visa-resource-name>, "error out"=w211:errorcluster)  [unwired: 11 in]
        n68 = call "Sensor.vi"("VISA resource name"=w217, "Channel (1)"=i32 ?, "error in (no error)"=w211) -> ("VISA resource name out"=w214:refnum<visa-resource-name>, "Resistance Reading"=w204:dbl, "error out"=w213:errorcluster)  [unwired: 8 in, 2 out]
        n69 = formula code="/*Used Chebychev polynomials fitting routine\nas described in Calibration Report Description \ndocument. For future use with other thermometer, \njust replace, in all the appropriate\nranges, the Chebychev coefficients (array 'A[i]'), \nthe lower and upper boundaries for Z (variables 'ZU' \nand 'ZL'), and the numberof polynomial terms or \nfit range (variable 'range'). This information is \nfound in the data file for the corresponding \nthermometer */\n\n/*Declare variables. Used same notation\nas Lakeshore Calibration Report Description*/\n\nfloat64 Z, ZL, ZU, X, T;\nfloat64 Tc[12], A[12];\nint range, i;\nZ=log(R);\n\n\n/*Fit range 3, for R between 122.7738 and\n379.0544*/\nif(R>122.7738 && R<=379.0544)\n{\nrange=7;\nZL= 2.06767500767592;\nZU= 2.62579727581576;\nX=((Z-ZL)-(ZU-Z))/(ZU-ZL);\nA[0]=5.89345488289531E+00;\nA[1]=-6.65662879806624E+00;\nA[2]=2.58839377481062E+00;\nA[3]=-7.79761085327563E-01;\nA[4]=1.81747664835559E-01;\nA[5]=-2.85948965899305E-02;\nA[6]=3.14756394066286E-04;\nA[7]=1.58182677797188E-03;\nA[8]=-1.62769128118703E-03;\n\nTc[0]=1;\nTc[1]=X;\nT=A[0]+A[1]*X;\n\nfor(i=2; i<=range; i++)\n{\nTc[i]=2*X*Tc[i-1]-Tc[i-2];\nT=T+Tc[i]*A[i];\n}\n}\n\n/*Fit range 2, for R between 59.7368 and\n122.7738*/\nif(R> 59.7368 && R<=122.7738)\n{\nrange=7;\nZL= 1.75200116332745;\nZU= 2.11435743095945;\nX=((Z-ZL)-(ZU-Z))/(ZU-ZL);\nA[0]=4.32234727947262E+01;\nA[1]=-3.81351999747578E+01;\nA[2]=7.81449116299263E+00;\nA[3]=-8.59375474039158E-01;\nA[4]= 1.00417492862823E-01;\nA[5]=1.74498449889679E-03;\nA[6]=-1.20713645610291E-02;\nA[7]=1.63447339264850E-03;\n\nTc[0]=1;\nTc[1]=X;\nT=A[0]+A[1]*X;\n\nfor(i=2; i<=range; i++)\n{\nTc[i]=2*X*Tc[i-1]-Tc[i-2];\nT=T+Tc[i]*A[i];\n}\n}\n\n/*Fit range 1, for R between 28.7437 and\n8273.0144*/\nif(R> 28.7437 && R<=59.7368)\n{\nrange=7;\nZL= 1.45494394005744;\nZU= 1.80316018562455;\nX=((Z-ZL)-(ZU-Z))/(ZU-ZL);\nA[0]=1.78354115735659E+02;\nA[1]=-1.26988903132178E+02;\nA[2]=2.11414551345279E+01;\nA[3]=-2.87039950284064E+00;\nA[4]= 6.30799574782896E-01;\nA[5]=-1.42209214015529E-01;\nA[6]=3.09622419372907E-02;\nA[7]=-9.63520999389506E-03;\n\nTc[0]=1;\nTc[1]=X;\nT=A[0]+A[1]*X;\n\nfor(i=2; i<=range; i++)\n{\nTc[i]=2*X*Tc[i-1]-Tc[i-2];\nT=T+Tc[i]*A[i];\n}\n}"("R"=w198) -> ("T"=w197:dbl)
        n70 = formula code="/*Used Chebychev polynomials fitting routine\nas described in Calibration Report Description \ndocument. For future use with other thermometer, \njust replace, in all the appropriate\nranges, the Chebychev coefficients (array 'A[i]'), \nthe lower and upper boundaries for Z (variables 'ZU' \nand 'ZL'), and the numberof polynomial terms or \nfit range (variable 'range'). This information is \nfound in the data file for the corresponding \nthermometer */\n\n/*Declare variables. Used same notation\nas Lakeshore Calibration Report Description*/\n\nfloat64 Z, ZL, ZU, X, T;\nfloat64 Tc[12], A[12];\nint range, i;\nZ=log(R);\n\n/*Fit range 4, for R between 27.8145 and\n55.2018*/\nif(R>=27.8145 && R<=55.2018)\n{\nrange=7;\nZL= 1.44074353015701;\nZU=1.76670659886134;\nX=((Z-ZL)-(ZU-Z))/(ZU-ZL);\nA[0]=1.82158062367373E+02;\nA[1]=-1.24663785394699E+02;\nA[2]= 1.99707471344437E+01;\nA[3]=-2.68638755066500E+00;\nA[4]=5.62902207096738E-01;\nA[5]= -1.04899492331528E-01;\nA[6]=1.47394426824740E-02;\nA[7]=-1.09663024188992E-02;\n\nTc[0]=1;\nTc[1]=X;\nT=A[0]+A[1]*X;\n\nfor(i=2; i<=range; i++)\n{\nTc[i]=2*X*Tc[i-1]-Tc[i-2];\nT=T+Tc[i]*A[i];\n}\n}\n\n/*Fit range 3, for R between 55.2018 and\n111.4842*/\nif(R>55.2018 && R<=111.4842)\n{\nrange=9;\nZL= 1.71936458773677;\nZU= 2.06940247551414;\nX=((Z-ZL)-(ZU-Z))/(ZU-ZL);\nA[0]=4.61222264729901E+01;\nA[1]=-4.01018177367225E+01;\nA[2]=8.04410401028361E+00;\nA[3]=-8.87825177741193E-01;\nA[4]= 9.46412812559081E-02;\nA[5]=1.14695723765652E-02;\nA[6]=-1.28476433375258E-02;\nA[7]=2.61003207902573E-03;\nA[8]=-1.62769128118703E-03;\nA[9]=2.14879733652881E-03;\n\nTc[0]=1;\nTc[1]=X;\nT=A[0]+A[1]*X;\n\nfor(i=2; i<=range; i++)\n{\nTc[i]=2*X*Tc[i-1]-Tc[i-2];\nT=T+Tc[i]*A[i];\n}\n}\n\n/*Fit range 2, for R between 111.4842 and\n313.6289*/\nif(R> 111.4842 && R<=313.6289)\n{\nrange=8;\nZL= 2.02806379707861;\nZU= 2.55512620740659;\nX=((Z-ZL)-(ZU-Z))/(ZU-ZL);\nA[0]=6.35009482366579E+00;\nA[1]=-7.12992063705802E+00;\nA[2]=2.72290509023981E+00;\nA[3]=-7.95127185574136E-01;\nA[4]= 1.75501651647015E-01;\nA[5]=-2.36820706103904E-02;\nA[6]=-1.48683367592906E-03;\nA[7]=2.20400453630561E-03;\nA[8]=-7.29658382785940E-04;\n\nTc[0]=1;\nTc[1]=X;\nT=A[0]+A[1]*X;\n\nfor(i=2; i<=range; i++)\n{\nTc[i]=2*X*Tc[i-1]-Tc[i-2];\nT=T+Tc[i]*A[i];\n}\n}\n\n/*Fit range 1, for R between 313.6289 and\n8273.0144*/\nif(R>  313.6289 && R<=8273.0144)\n{\nrange=11;\nZL= 2.43768275202674;\nZU= 4.08120684160154;\nX=((Z-ZL)-(ZU-Z))/(ZU-ZL);\nA[0]=5.67750174822212E-01;\nA[1]=-7.48399352555430E-01;\nA[2]=3.88178435547519E-01;\nA[3]=-1.77340445603059E-01;\nA[4]= 7.34297995027544E-02;\nA[5]=-2.89170333461975E-02;\nA[6]=1.12452775189607E-02;\nA[7]=-3.77083878348011E-03;\nA[8]=1.58754722583042E-03;\nA[9]=-1.76346768933995E-04;\nA[10]=4.11858083918786E-04;\nA[11]=3.67394984257076E-04;\n\nTc[0]=1;\nTc[1]=X;\nT=A[0]+A[1]*X;\n\nfor(i=2; i<=range; i++)\n{\nTc[i]=2*X*Tc[i-1]-Tc[i-2];\nT=T+Tc[i]*A[i];\n}\n}"("R"=w208) -> ("T"=w206:dbl)
        n71 = formula code="/*Used Chebychev polynomials fitting routine\nas described in Calibration Report Description \ndocument. For future use with other thermometer, \njust replace, in all the appropriate\nranges, the Chebychev coefficients (array 'A[i]'), \nthe lower and upper boundaries for Z (variables 'ZU' \nand 'ZL'), and the numberof polynomial terms or \nfit range (variable 'range'). This information is \nfound in the data file for the corresponding \nthermometer */\n\n/*Declare variables. Used same notation\nas Lakeshore Calibration Report Description*/\n\nfloat64 Z, ZL, ZU, X, T;\nfloat64 Tc[12], A[12];\nint range, i;\nZ=log(R);\n\n/*Fit range 4, for R between 27.8145 and\n55.2018*/\nif(R>=27.8145 && R<=55.2018)\n{\nrange=7;\nZL= 1.44074353015701;\nZU=1.76670659886134;\nX=((Z-ZL)-(ZU-Z))/(ZU-ZL);\nA[0]=1.82158062367373E+02;\nA[1]=-1.24663785394699E+02;\nA[2]= 1.99707471344437E+01;\nA[3]=-2.68638755066500E+00;\nA[4]=5.62902207096738E-01;\nA[5]= -1.04899492331528E-01;\nA[6]=1.47394426824740E-02;\nA[7]=-1.09663024188992E-02;\n\nTc[0]=1;\nTc[1]=X;\nT=A[0]+A[1]*X;\n\nfor(i=2; i<=range; i++)\n{\nTc[i]=2*X*Tc[i-1]-Tc[i-2];\nT=T+Tc[i]*A[i];\n}\n}\n\n/*Fit range 3, for R between 55.2018 and\n111.4842*/\nif(R>55.2018 && R<=111.4842)\n{\nrange=9;\nZL= 1.71936458773677;\nZU= 2.06940247551414;\nX=((Z-ZL)-(ZU-Z))/(ZU-ZL);\nA[0]=4.61222264729901E+01;\nA[1]=-4.01018177367225E+01;\nA[2]=8.04410401028361E+00;\nA[3]=-8.87825177741193E-01;\nA[4]= 9.46412812559081E-02;\nA[5]=1.14695723765652E-02;\nA[6]=-1.28476433375258E-02;\nA[7]=2.61003207902573E-03;\nA[8]=-1.62769128118703E-03;\nA[9]=2.14879733652881E-03;\n\nTc[0]=1;\nTc[1]=X;\nT=A[0]+A[1]*X;\n\nfor(i=2; i<=range; i++)\n{\nTc[i]=2*X*Tc[i-1]-Tc[i-2];\nT=T+Tc[i]*A[i];\n}\n}\n\n/*Fit range 2, for R between 111.4842 and\n313.6289*/\nif(R> 111.4842 && R<=313.6289)\n{\nrange=8;\nZL= 2.02806379707861;\nZU= 2.55512620740659;\nX=((Z-ZL)-(ZU-Z))/(ZU-ZL);\nA[0]=6.35009482366579E+00;\nA[1]=-7.12992063705802E+00;\nA[2]=2.72290509023981E+00;\nA[3]=-7.95127185574136E-01;\nA[4]= 1.75501651647015E-01;\nA[5]=-2.36820706103904E-02;\nA[6]=-1.48683367592906E-03;\nA[7]=2.20400453630561E-03;\nA[8]=-7.29658382785940E-04;\n\nTc[0]=1;\nTc[1]=X;\nT=A[0]+A[1]*X;\n\nfor(i=2; i<=range; i++)\n{\nTc[i]=2*X*Tc[i-1]-Tc[i-2];\nT=T+Tc[i]*A[i];\n}\n}\n\n/*Fit range 1, for R between 313.6289 and\n8273.0144*/\nif(R>  313.6289 && R<=8273.0144)\n{\nrange=11;\nZL= 2.43768275202674;\nZU= 4.08120684160154;\nX=((Z-ZL)-(ZU-Z))/(ZU-ZL);\nA[0]=5.67750174822212E-01;\nA[1]=-7.48399352555430E-01;\nA[2]=3.88178435547519E-01;\nA[3]=-1.77340445603059E-01;\nA[4]= 7.34297995027544E-02;\nA[5]=-2.89170333461975E-02;\nA[6]=1.12452775189607E-02;\nA[7]=-3.77083878348011E-03;\nA[8]=1.58754722583042E-03;\nA[9]=-1.76346768933995E-04;\nA[10]=4.11858083918786E-04;\nA[11]=3.67394984257076E-04;\n\nTc[0]=1;\nTc[1]=X;\nT=A[0]+A[1]*X;\n\nfor(i=2; i<=range; i++)\n{\nTc[i]=2*X*Tc[i-1]-Tc[i-2];\nT=T+Tc[i]*A[i];\n}\n}"("R"=w204) -> ("T"=w202:dbl)
        n72 = Number To Exponential String(number=w198) -> (E-format string=w210:string)  [unwired: 3 in]
        n73 = Number To Exponential String(number=w197) -> (E-format string=w209:string)  [unwired: 3 in]
        n74 = Number To Exponential String(number=w208) -> (E-format string=w207:string)  [unwired: 3 in]
        n75 = Number To Exponential String(number=w206) -> (E-format string=w205:string)  [unwired: 3 in]
        n76 = Number To Exponential String(number=w204) -> (E-format string=w203:string)  [unwired: 3 in]
        n77 = Number To Exponential String(number=w202) -> (E-format string=w200:string)  [unwired: 3 in]
        n78 = Concatenate Strings(w201, w210, w201, w209, w201, w207, w201, w205, w201, w203, w201, w200) -> (w199:string)
      }
    }
    "Cernox Temperature 3" <- w30
    "Cernox Temperature 1" <- w32
    "Cernox Temperature 2" <- w31
    n79 = Get Date/Time In Seconds() -> (seconds since 1Jan1904=w63:timestamp)
    n80 = Format Date/Time String(seconds (now)=w63) -> (date/time string=w43:string)  [unwired: 2 in]
    n81 = call "XY- Graph As Chart.vi"("Y-Value"=w32, "X- Value"=w36) -> ("XY Graph"=→"Channel 1":cluster{dbl[], dbl[]})  [unwired: 3 in]
    n82 = Open/Create/Replace File(file path (use dialog)="File Path", operation (0:open)=T1 ?) -> (refnum out=w60:refnum<file>, error out=w59:errorcluster)  [unwired: 4 in, 1 out]
    n83 = call "XY- Graph As Chart.vi"("Y-Value"=w31, "X- Value"=w36) -> ("XY Graph"=→"Channel 2":cluster{dbl[], dbl[]})  [unwired: 3 in]
    n84 = call "XY- Graph As Chart.vi"("Y-Value"=w30, "X- Value"=w36) -> ("XY Graph"=→"Channel 3":cluster{dbl[], dbl[]})  [unwired: 3 in]
    n85 = Concatenate Strings(w43, w29, string ?) -> (w42:string)
    n86 = Set File Position(refnum=w60, error in=w59) -> (refnum out=w58:refnum<file>, error out=w57:errorcluster)  [unwired: 2 in]
    n87 = Write to Text File(file (use dialog)=w58, text=w42, error in=w57) -> (refnum out=w56:refnum<file>, error out=w55:errorcluster)  [unwired: 1 in, 1 out]
  }
  n88 = Close File(refnum=w17, error in=w16) -> ()  [unwired: 2 out]
  n89 = call "Close.vi"("VISA resource name"=w4, "error in (no error)"=w3) -> ()  [unwired: 13 in, 1 out]
  n90 = call "fl884x Close.vi"("error in (no error)"=w18, "VISA resource name"=w15) -> ()  [unwired: 9 in, 1 out]
